vi "HDF5 append data (DBL 1D).vi"(8 "error in (no error)":errorcluster, 10 "data":dbl[](array[numeric]), 11 "dset in":i32) -> (0 "error out":errorcluster, 3 "ref out":i32)   [LabVIEW 2012]
uses:
  <vilib>/addons/h5labview2/base/H5Equery.vi
  <vilib>/addons/h5labview2/dataset/H5Dwrite.llb/H5Dwrite.xnode
  <vilib>/addons/h5labview2/dataset/H5D.lvlib
  <vilib>/addons/h5labview2/space/H5S.lvlib
  <vilib>/addons/h5labview2/h5labview32.dll
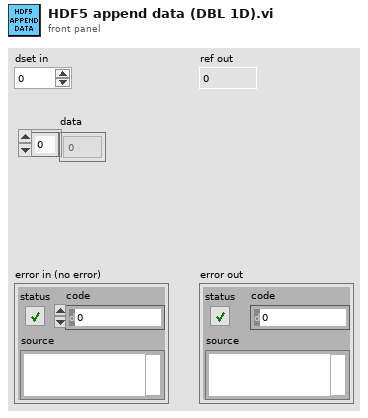
[diagram p1: front panel]
types:
  T1 = typedef "hid_t.ctl" = i32
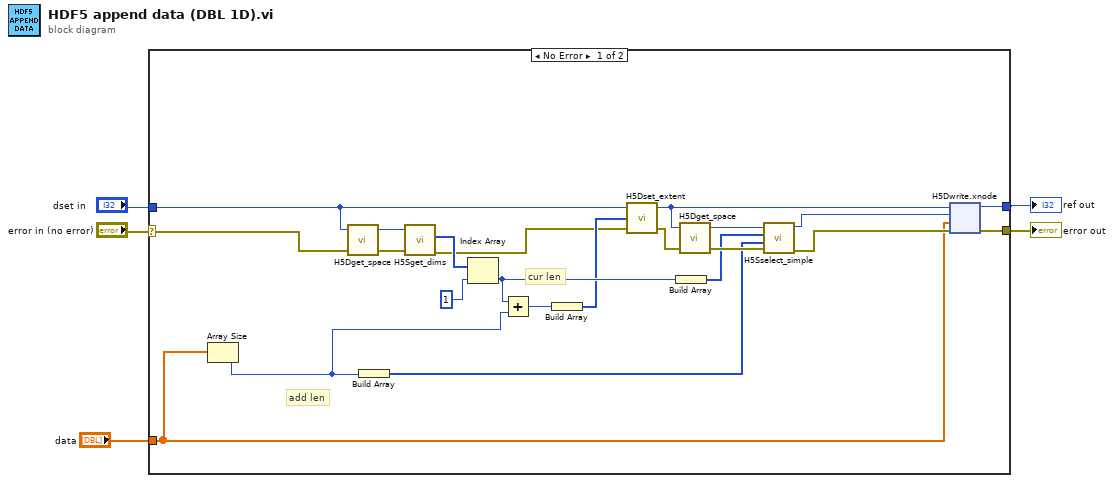
[diagram p0: block diagram]
diagram:
  n1 = case shown="No Error" "error in (no error)" {
    selector: "error in (no error)" -> [w16 w45]
    tunnel: [w27 w45] -> w5
    tunnel: [w26 w46] -> w4
    tunnel: "dset in" -> [w21 w46]
    tunnel: "data" -> [w18 _]
    frame No Error {
      # "cur len"
      # "add len"
      n2 = Array Size(array=w18) -> (size(s)=w11:i32)
      n3 = call <vilib>:"H5Dget_space.vi"("error in (no error)"=w16, "ref in"=w21) -> ("error out"=w23:errorcluster, "space out"=w22:i32)  [unwired: 2 in]
      n4 = Build Array(w11) -> (w6:i32[])
      n5 = call <vilib>:"H5Sget_dims.vi"("error in (no error)"=w23, "space in"=w22) -> ("error out"=w8:errorcluster, "dims"=w14:u32[])  [unwired: 2 in, 2 out]
      n6 = Index Array(array=w14, index=1) -> (element=w13:u32)
      n7 = Add(x=w13, y=w11) -> (x+y=w10:u32)
      n8 = Build Array(w10) -> (w9:u32[])
      n9 = call <vilib>:"H5Dset_extent.vi"("error in (no error)"=w8, "new size"=w9, "dset in"=w21) -> ("error out"=w7:errorcluster, "dset out"=w17:i32)  [unwired: 1 in]
      n10 = Build Array(w13) -> (w12:u32[])
      n11 = call <vilib>:"H5Dget_space.vi"("error in (no error)"=w7, "ref in"=w17) -> ("error out"=w20:errorcluster, "space out"=w19:i32)  [unwired: 2 in]
      n12 = call <vilib>:"H5Sselect_simple.vi"("error in (no error)"=w20, "count"=w6, "start"=w12, "space in"=w19) -> ("error out"=w25:errorcluster, "space out"=w24:T1)  [unwired: 2 in]
      n13 = xnode "H5Dwrite.xnode"("error in (no error)"=w25, "data"=w18, "file space"=w24, "ref in"=w17) -> ("error out"=w27:errorcluster, "ref out"=w26:i32)  [unwired: 3 in, 1 out]
    }
    frame Error {
    }
  }
  "error out" <- w5
  "ref out" <- w4
